vi "Ethernet Writer Modified.vi"() -> ()   [LabVIEW 2022 SP3]
doc: "This example creates a frame output stream session and allows the user to write Ethernet frames."
uses:
  <vilib>/xnet/xnet.llb/XNET Frame Ethernet.ctl
  <vilib>/xnet/xnet.llb/XNET Frame Type Ethernet.ctl
  Program Files/National Instruments/LabVIEW 2022/examples/nixnet/projects/NI-XNET Ethernet/subVI/Ethernet/Controls/Ethernet Header.ctl
  Program Files/National Instruments/LabVIEW 2022/examples/nixnet/projects/NI-XNET Ethernet/subVI/Ethernet/Controls/VLAN Tag.ctl
  <vilib>/xnet/xnet.llb/XNET Create Session (Frame Output Stream).vi
  <vilib>/xnet/xnet.llb/XNET Write (Frame Ethernet).vi
  Program Files/National Instruments/LabVIEW 2022/examples/nixnet/projects/NI-XNET Ethernet/subVI/Ethernet.lvlib
  <resource>/objmgr/xnet.rc
panel:
  out "current time":timestamp
  out "Port State":u32(ring)=3 items=["Disabled"=3, "Master"=6, "Passive"=7, "Slave"=9]
  out "Number of Frames Sent":u32
  in  "priority":u8=3
  in  "VID":u16=2
  in  "Ethertype":u16=34997 format="%.0x"
  in  "Has VLAN Tag":bool=TRUE
  in  "destination MAC address":cluster{u8, u8, u8, u8, u8, u8}={255, 255, 255, 255, 255, 255} {"?" format="%.0x"; "?" format="%.0x"; "?" format="%.0x"; "?" format="%.0x"; "?" format="%.0x"; "?" format="%.0x"}
  in  "payload":string="\u0000\u0001\u0002\u0003\u0004\u0005\u0006\u0007\b\t\n\u000b\f\r\u000e\u000f\u0010\u0011\u0012\u0013\u0014\u0015\u0016\u0017\u0018\u0019\u001a\u001b\u001c\u001d\u001e\u001f !\"#$%&'()*+,-./0123456789:;<=>?@ABCDEFGHIJKLMNOPQRSTUVWXYZ[\\]^_`abc"
  in  "Write Frame":bool
  in  "Stop":bool
  in  "Interface":refnum<k21>="ENET1"
  # "Overview: Demonstrates writing frames on an Ethernet frame output stream.\nRequirements: LabVIEW, NI-XNET\nInstructions:\n1. Select an interface.\n2. Check that the PHY State of the selected interface is compatible with the interface it is connected to. For example, if the connected interface is in \"Master\" mode, the interface will need to be configured to \"Slave\". Use NI MAX to change the PHY State setting.\n3. Check that the Port Mode of the selected interface is configured to \"Direct\". Use NI MAX to change the Port Mode setting.\n4. Run the VI.\n5. The controls enclosed in the frame on the front panel represent fields of an Ethernet frame \nto write. Fill out the destination MAC address, VLAN tag information, Ethertype, and payload \nas needed. Note: by default, the source MAC address will automatically be filled in by XNET.\n6. Click Write Frame to write the Ethernet frame. \n7. When finished, click the Stop button."
  # "Note: VID and priority are \nonly encoded when Has \nVLAN Tag is true."
  # "Note: padding bytes are automatically added if the frame data is less than 60 bytes."
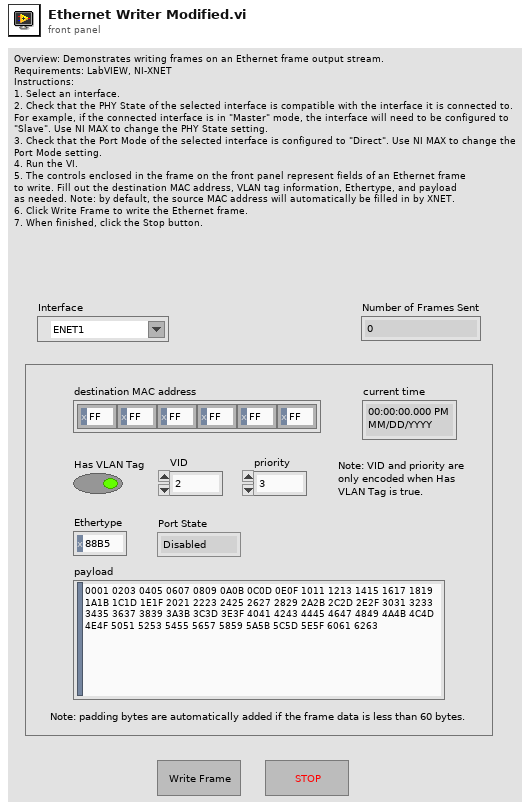
[diagram p1: front panel]
types:
  T1 = typedef "Ethernet.lvlib/VLAN Tag.ctl" = cluster{"TPID":u16, "priority":u8, "DEI":bool, "VID":u16}
  T2 = typedef "Ethernet.lvlib/Ethernet Header.ctl" = cluster{"destination MAC address":cluster{u8, u8, u8, u8, u8, u8}, "source MAC address":cluster{u8, u8, u8, u8, u8, u8}, "Has VLAN Tag":bool, "VLAN Tag":T1, "Ethertype":u16}
  T3 = typedef "XNET Frame Ethernet.ctl" = cluster{"local timestamp":timestamp, "network timestamp":timestamp, "frame data":u8[], "fcs":u32, "type":T4, "network synced?":bool, "receive?":bool, "transmit?":bool, "error?":bool}
  T4 = typedef "XNET Frame Type Ethernet.ctl" = u16
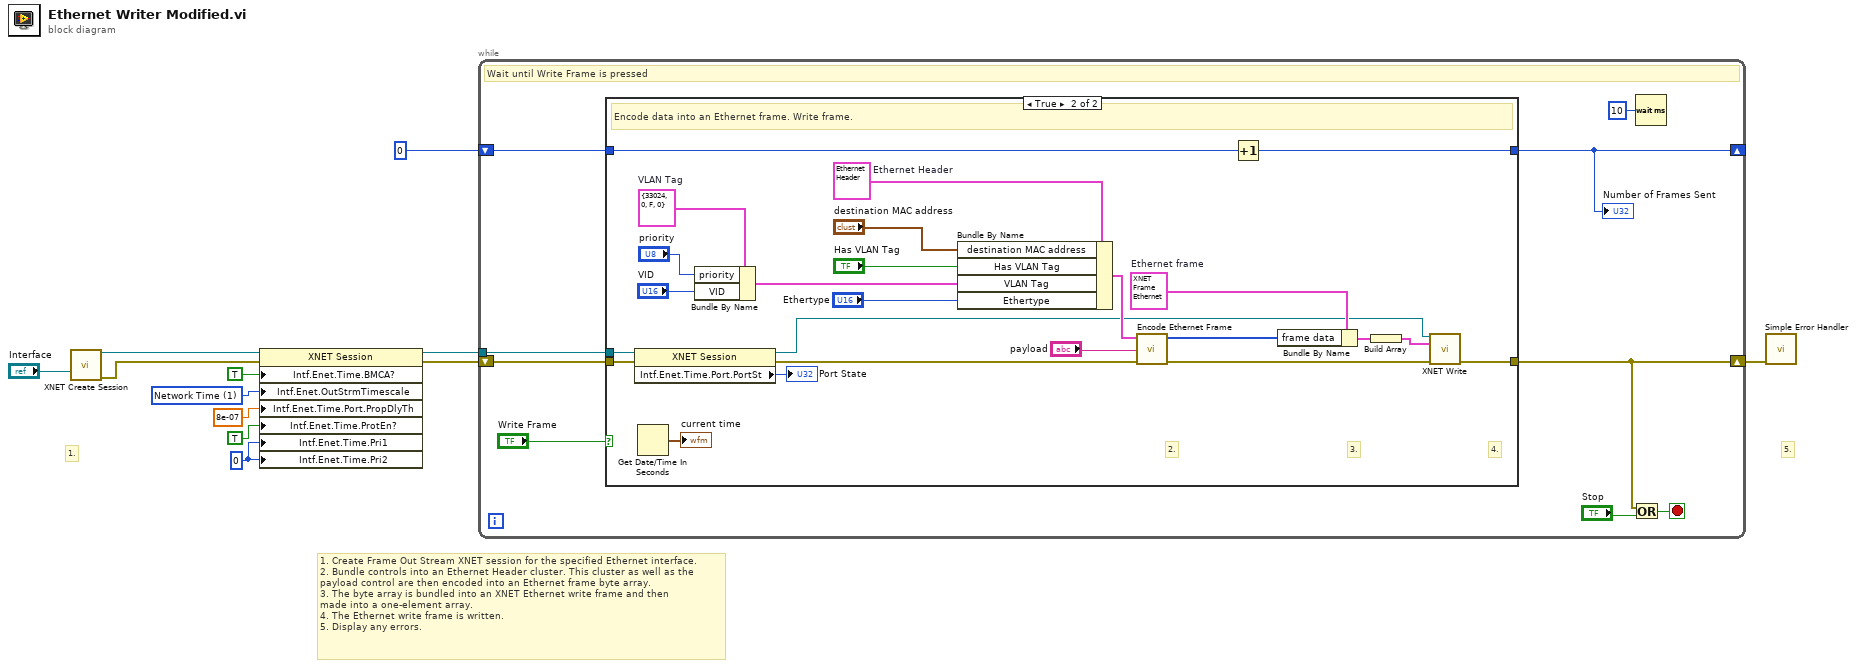
[diagram p0: block diagram]
diagram:
  w4 = u32 1 items=["Local Time", "Network Time"] ("Interface:Ethernet:Output Stream Timescale")
  w1 = u32 0 ("Interface:Ethernet:Time Sync:Priority1")
  # "1. Create Frame Out Stream XNET session for the specified Ethernet interface.\n2. Bundle controls into an Ethernet Header cluster. This cluster as well as the\npayload control are then encoded into an Ethernet frame byte array.\n3. The byte array is bundled into an XNET Ethernet write frame and then\nmade into a one-element array.\n4. The Ethernet write frame is written.\n5. Display any errors."
  # "5."
  # "1."
  n1 = call-poly <vilib>:"XNET Create Session.vi"("interface"="Interface") -> ("session out"=w9:refnum<k21>, "error out"=w8:errorcluster)  [unwired: 13 in]
  n2 = property class="XNET Session"(reference=w9, error in=w8, "Intf.Enet.Time.BMCA?"=TRUE ("Interface:Ethernet:Time Sync:Protocol Enabled?"), "Intf.Enet.OutStrmTimescale"=w4, "Intf.Enet.Time.Port.PropDlyTh"=8e-07 ("Propagation Delay Threshold (s)"), "Intf.Enet.Time.ProtEn?"=TRUE ("Interface:Ethernet:Time Sync:Protocol Enabled?"), "Intf.Enet.Time.Pri1"=w1, "Intf.Enet.Time.Pri2"=w1) -> (reference out=w6:refnum<k21>, error out=w7:errorcluster)
  n3 = while {
    shift-right: [w17] -> w11
    shift-left: w7 -> [w19]
    tunnel: w6 -> [w20]
    shift-right: [w13] -> _
    shift-left: u32 0 -> [w14]
    stop <- w16 stop-if-true
    # "Wait until Write Frame is pressed"
    n4 = case shown="True" "Write Frame" {
      tunnel: w20 -> [_ w30]
      tunnel: w19 -> [w23 w29]
      tunnel: [w23 w39] -> w17
      tunnel: w14 -> [w22 w33]
      tunnel: [w22 w32] -> w13
      frame False {
      }
      frame True {
        w37 = T1 {"TPID"=33024, "priority"=0, "DEI"=FALSE, "VID"=0}  # VLAN Tag
        w38 = T2 {"destination MAC address"={0, 0, 0, 0, 0, 0}, "source MAC address"={0, 0, 0, 0, 0, 0}, "Has VLAN Tag"=FALSE, "VLAN Tag"={"TPID"=33024, "priority"=0, "DEI"=FALSE, "VID"=0}, "Ethertype"=0}  # Ethernet Header
        w42 = T3 {"local timestamp"=timestamp(0 s since 1904-01-01), "network timestamp"=timestamp(0 s since 1904-01-01), "frame data"=[], "fcs"=0, "type"=0, "network synced?"=FALSE, "receive?"=FALSE, "transmit?"=FALSE, "error?"=FALSE}  # Ethernet frame
        # "4."
        # "3."
        # "2."
        # "Encode data into an Ethernet frame. Write frame."
        n5 = property class="XNET Session"(reference=w30, error in=w29) -> (reference out=w25:refnum<k21>, error out=w28:errorcluster, "Intf.Enet.Time.Port.PortSt"=→"Port State":u32)
        n6 = Get Date/Time In Seconds() -> (seconds since 1Jan1904=→"current time":timestamp)
        n7 = Bundle By Name(cluster=w37, "priority"="priority", "VID"="VID") -> (w36:T1)
        n8 = Bundle By Name(cluster=w38, "destination MAC address"="destination MAC address", "Has VLAN Tag"="Has VLAN Tag", "VLAN Tag"=w36, "Ethertype"="Ethertype") -> (w26:T2)
        n9 = call "Encode Ethernet Frame.vi"("error in (no error)"=w28, "payload"="payload", "Ethernet Header"=w26) -> ("error out"=w43:errorcluster, "frame data"=w41:u8[])  [unwired: 7 in]
        n10 = Increment(x=w33) -> (x+1=w32:u32)
        n11 = Bundle By Name(cluster=w42, "frame data"=w41) -> (w40:T3)
        n12 = Build Array(w40) -> (w24:T3[])
        n13 = call-poly <vilib>:"XNET Write.vi"("session in"=w25, "data"=w24, "error in (no error)"=w43) -> ("error out"=w39:errorcluster)  [unwired: 11 in, 1 out]
      }
    }
    "Number of Frames Sent" <- w13
    n14 = Or(x=w17, y="Stop") -> (x .or. y?=w16:bool)
    n15 = Wait (ms)(milliseconds to wait=u32 10) -> ()  [unwired: 1 out]
  }
  n16 = call <vilib>:"Simple Error Handler.vi"("error in (no error)"=w11) -> ()  [unwired: 4 in, 5 out]
